vi "Key Down.vi"(8 "error in (no error)":errorcluster, 10 "delay in ms (80)":u32=80, 11 "Virtual Key":u8(ring)=65) -> (0 "error out":errorcluster)   [LabVIEW 2017]
doc: "call keybd_event drom user32.dll library to generate the key down event on desired key"
uses:
  3e1baad8-e73b-4a13-910d-5cdf89a6fe8a.vi
  User32.dll
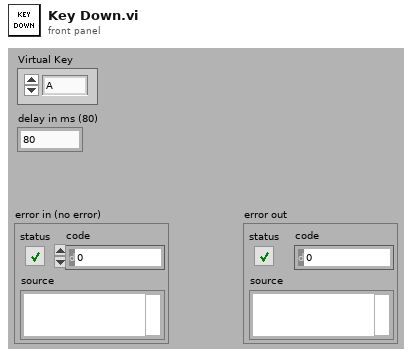
[diagram p1: front panel]
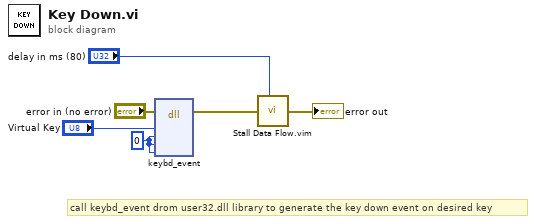
[diagram p0: block diagram]
diagram:
  w6 = u8 0 ("bScan")
  # "call keybd_event drom user32.dll library to generate the key down event on desired key"
  n1 = dll-call lib="user32.dll" fn="keybd_event"(error in="error in (no error)", "bVk"="Virtual Key", "bScan"=w6, "dwFlags"=w6, "dwExtraInfo"=w6) -> (error out=w3:errorcluster)  [unwired: 7 in, 1 out]
  n2 = call "Stall Data Flow.vim"("value in"=w3, "milliseconds to wait"="delay in ms (80)") -> ("value out"=→"error out":errorcluster)  [unwired: 1 out]
